vi "Write Client ID.vi"(8 "error in":errorcluster, 10 "Client ID":string, 11 "Launch Client in":refnum<class "Launch Client.lvclass">) -> (0 "error out":errorcluster, 3 "Launch Client out":refnum<class "Launch Client.lvclass">)   [LabVIEW 2014, in "Launch Client.lvclass"]
uses:
  Launch Client.lvclass
  Launch Client.lvclass/Launch Client.ctl
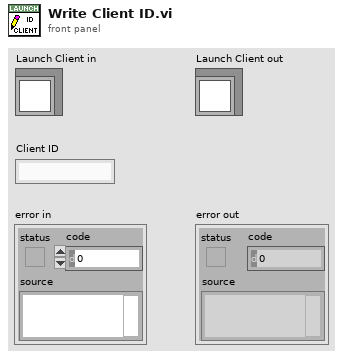
[diagram p1: front panel]
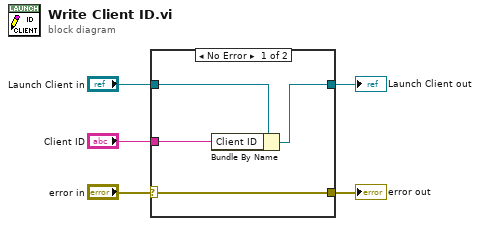
[diagram p0: block diagram]
diagram:
  n1 = case shown="No Error" "error in" {
    selector: "error in" -> [w9 w10]
    tunnel: [w9 w10] -> w4
    tunnel: [w7 w11] -> w2
    tunnel: "Launch Client in" -> [w8 w11]
    tunnel: "Client ID" -> [w6 _]
    frame No Error {
      n2 = Bundle By Name(cluster=w8, "Client ID"=w6) -> (w7:refnum<class "Launch Client.lvclass">)
    }
    frame Error {
    }
  }
  "error out" <- w4
  "Launch Client out" <- w2
